vi "Router - Get Data from Table.vi"(8 "error in (no error)":errorcluster) -> (0 "error out":errorcluster)   [LabVIEW 2016]
uses:
  PXImc Router/Controls/Table Index-Size.ctl
  PXImc Router/PXImc Router.lvlib
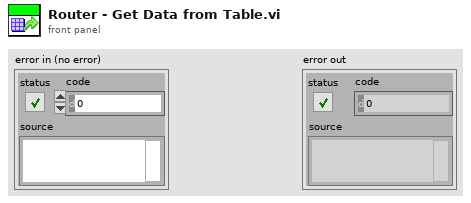
[diagram p1: front panel]
types:
  T1 = typedef "PXImc Router.lvlib/Table Index-Size.ctl" = cluster{"Index":u32, "Size":u32}
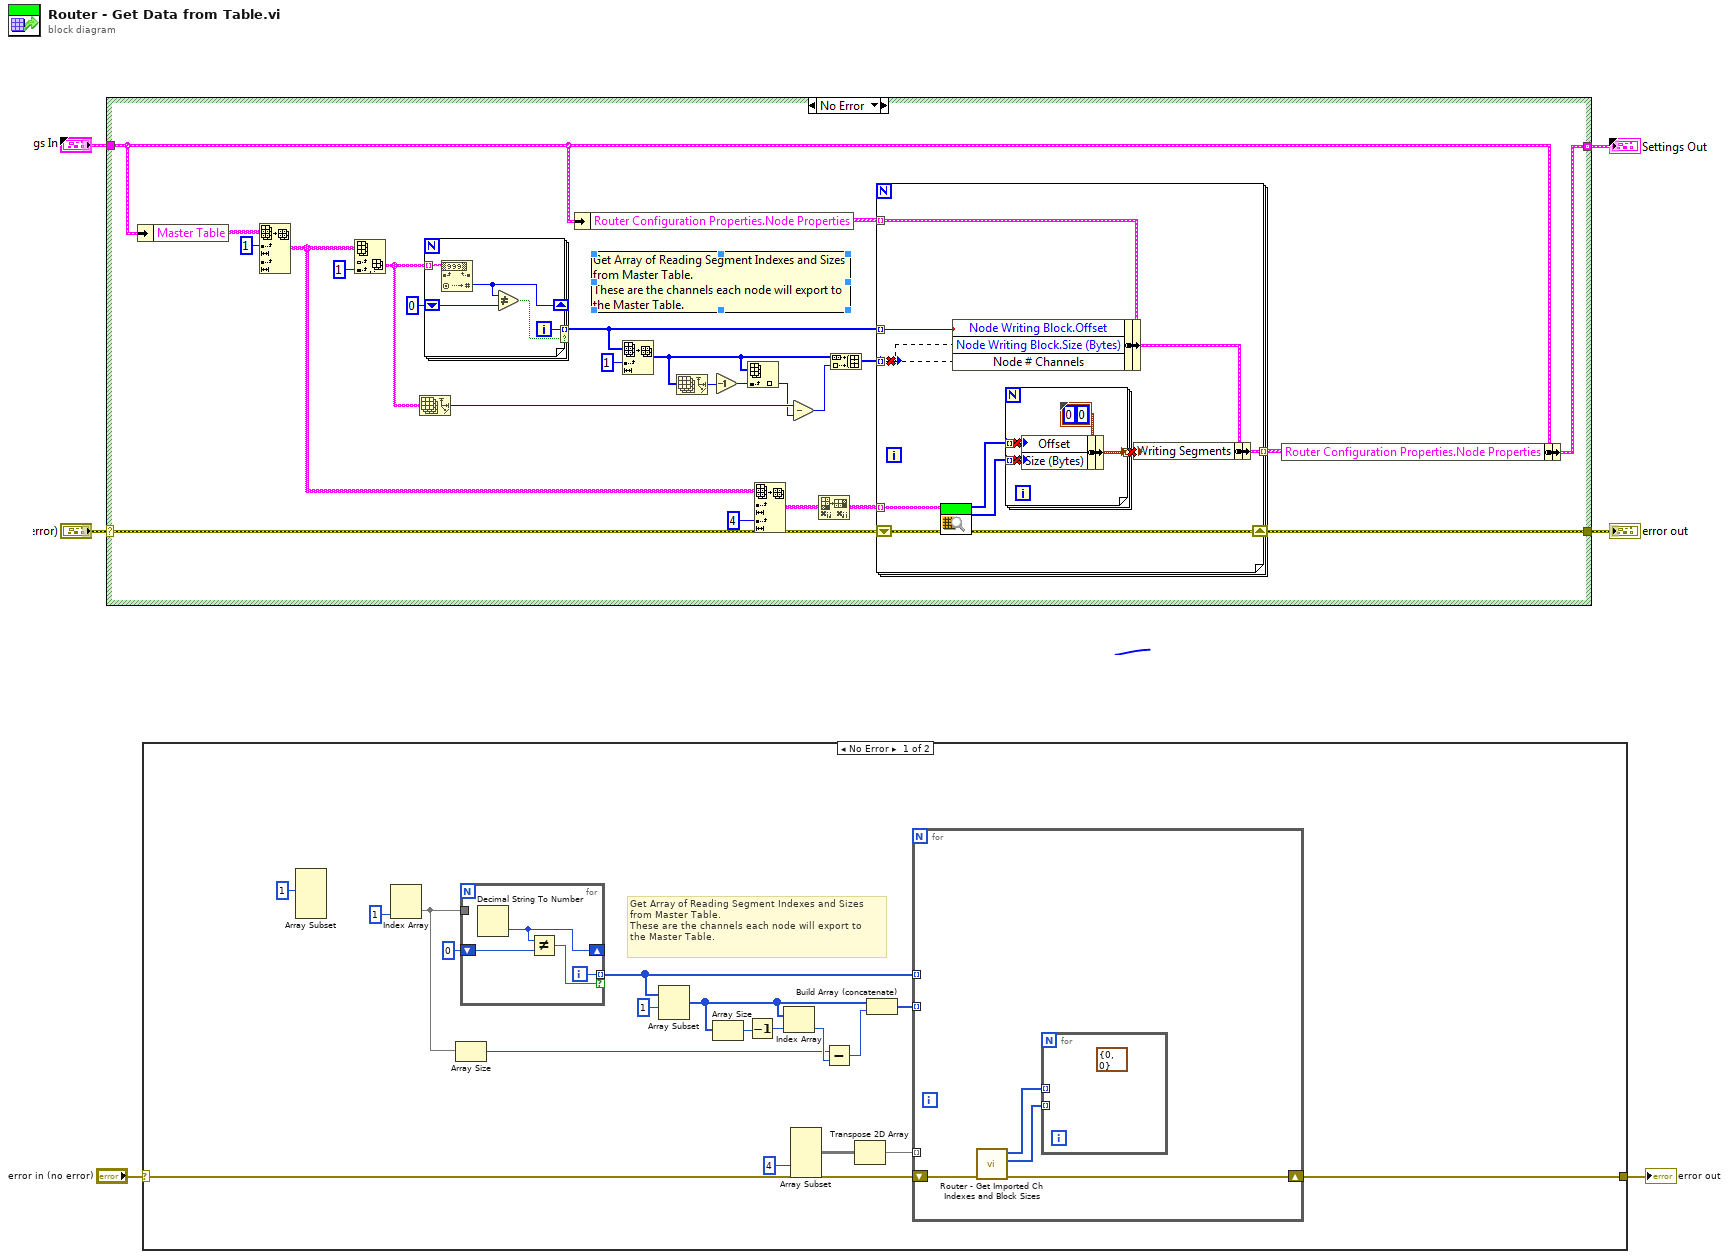
[diagram p0: block diagram]
diagram:
  n1 = case shown="No Error" "error in (no error)" {
    selector: "error in (no error)" -> [w4 w29]
    tunnel: [w3 w29] -> w1
    frame No Error {
      # "Get Array of Reading Segment Indexes and Sizes \nfrom Master Table.\nThese are the channels each node will export to\nthe Master Table."
      n2 = Array Subset(index (row)=1 ("index")) -> ()  [unwired: 4 in, 1 out]
      n3 = Index Array(index (col)=1 ("disabled index (col)")) -> (element=w8)  [unwired: 2 in]
      n4 = Array Size(array=w8) -> (size(s)=w13:i32)
      n5 = for {
        tunnel: w8 -> [_]
        shift-right: [w25] -> _
        shift-left: 0 -> [w28]
        tunnel: [w26] -> w9 mode=indexing if=w27
        i -> [w26]
        n6 = Decimal String To Number() -> (number=w25:i32)  [unwired: 3 in, 1 out]
        n7 = Not Equal?(x=w25, y=w28) -> (x != y?=w27:bool)
      }
      n8 = Array Subset(array=w9, index=1) -> (w17:i32[])  [unwired: 1 in]
      n9 = Array Size(array=w17) -> (size(s)=w11:i32)
      n10 = Decrement(x=w11) -> (x-1=w12:i32)
      n11 = Index Array(array=w17, index=w12) -> (element=w14:i32)
      n12 = Array Subset(index (col)=4 ("index")) -> (w19:void[][])  [unwired: 4 in]
      n13 = Subtract(x=w13, y=w14) -> (x-y=w15:i32)
      n14 = Transpose 2D Array(2D array=w19) -> (transposed array=w20:void[][])
      n15 = Build Array (concatenate)(w17, w15) -> (w16:i32[])
      n16 = for {
        tunnel: w9 -> [_] mode=indexing
        tunnel: w16 -> [_] mode=indexing
        tunnel: w20 -> [_] mode=indexing
        shift-right: [w21] -> w3
        shift-left: w4 -> [w22]
        n17 = call "Router - Get Imported Ch Indexes and Block Sizes.vi"("error in (no error)"=w22) -> ("error out"=w21:errorcluster, "Block Sizes"=w23:i32[], "Indexes"=w24:i32[])  [unwired: 8 in]
        n18 = for {
          tunnel: w23 -> [_] mode=indexing
          tunnel: w24 -> [_] mode=indexing
          (unwired) T1 {"Index"=0, "Size"=0} ("Table Index-Size")
        }
      }
    }
    frame Error {
    }
  }
  "error out" <- w1
